vi "Browse for Sequence.vi"(8 "error in (no error)":errorcluster, 10 "Caption (Browse for/Select concatenated)":string, 11 "Browse start path":path) -> (0 "error out":errorcluster, 1 "Cancelled?":bool, 3 "File Path out":path)   [LabVIEW 2020, in "Sequencer.lvlib"]
doc: "Save the uncompiled sequence to a sequence file."
uses:
  Sequencer.lvlib
panel:
  in  "Cancel":bool
  in  "OK":bool
  in  "File Path Control":path
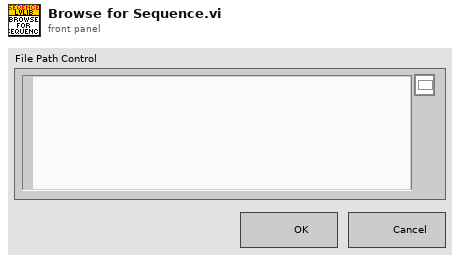
[diagram p1: front panel]
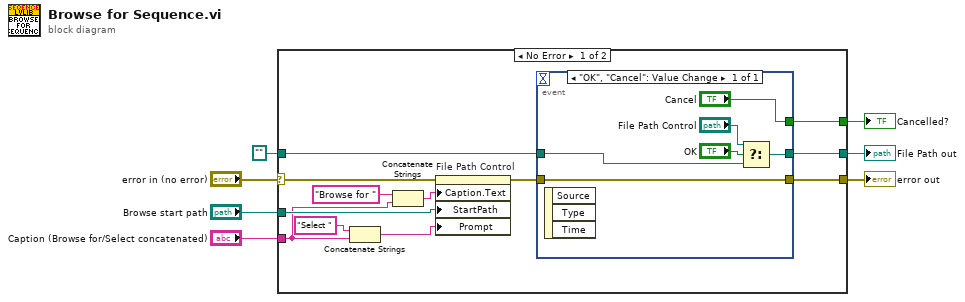
[diagram p0: block diagram]
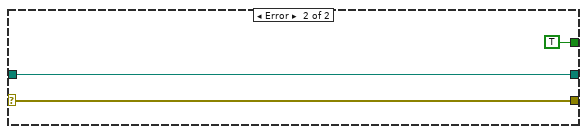
[diagram p2: hidden frame]
diagram:
  n1 = case shown="No Error" "error in (no error)" {
    selector: "error in (no error)" -> [w13 w28]
    tunnel: [w11 w28] -> w7
    tunnel: "Browse start path" -> [w17 _]
    tunnel: "Caption (Browse for/Select concatenated)" -> [w15 _]
    tunnel: [w10 w26] -> w3
    tunnel: [w9 TRUE ("Cancel")] -> w1
    tunnel: path "" -> [w8 w26]
    frame No Error {
      n2 = Concatenate Strings("Select " ("string"), w15) -> (w14:string)
      n3 = Concatenate Strings("Browse for " ("string"), w15) -> (w18:string)
      n4 = property on="File Path Control" class="Path"(error in=w13, "Caption.Text"=w18, "StartPath"=w17, "Prompt"=w14) -> (error out=w12:errorcluster)  [unwired: 1 in, 1 out]
      n5 = event shown="[0] \"OK\", \"Cancel\": Value Change" {
        selector: _ -> [_]
        dyn-events: _ -> [_]
        timeout: _ -> [_]
        tunnel: w12 -> [w25]
        tunnel: [w25] -> w11
        tunnel: [w22] -> w10
        tunnel: ["Cancel"] -> w9
        tunnel: w8 -> [w20]
        event "OK", "Cancel": Value Change {
          n6 = event-data() -> ()  [unwired: 1 in, 3 out]
          n7 = Select(t="File Path Control", s="OK", f=w20) -> (s? t:f=w22:path)
        }
      }
    }
    frame Error {
    }
  }
  "error out" <- w7
  "File Path out" <- w3
  "Cancelled?" <- w1
